vi "Read DI.vi"(6 "wait for reply (T)":bool=TRUE, 8 "error in":errorcluster, 11 "Module ID":i32=-1) -> (0 "error out":errorcluster, 1 "timed out?":bool, 3 "DI":bool[](array[boolean]))   [LabVIEW 2020, in "NI DAQ Aug 25.lvlib"]
doc: "Reads single or multiple DIs."
uses:
  NI DAQ Aug 25.lvlib
  Read DI Argument--cluster.ctl
  Read DI (Reply Payload)--cluster.ctl
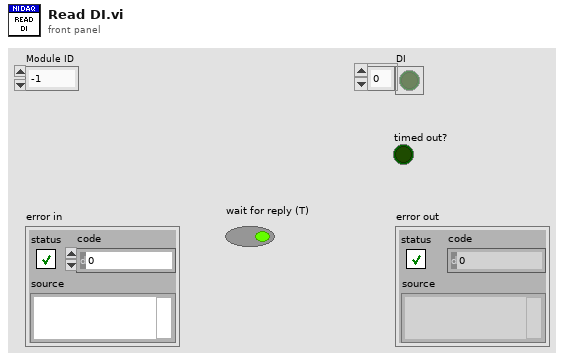
[diagram p1: front panel]
types:
  T1 = typedef "NI DAQ Aug 25.lvlib/Read DI Argument--cluster.ctl" = cluster{"Module ID":i32, "Boolean":bool, "Wait Notifier":refnum<notifier>, "wait for reply":bool}
  T2 = typedef "NI DAQ Aug 25.lvlib/Request Events--cluster.ctl" = cluster{"Stop Module":refnum<user-event>, "Show Panel":refnum<user-event>, "Hide Panel":refnum<user-event>, "Show Diagram":refnum<user-event>, "Get Module Execution Status":refnum<user-event>, "Draw FP in subpanel":refnum<user-event>, "Remove from subpanel":refnum<user-event>, "Set device name":refnum<user-event>, "Write DO":refnum<user-event>, "Create DO channel":refnum<user-event>, "Create DI channel":refnum<user-event>, "Read DI":refnum<user-event>}
  T3 = typedef "NI DAQ Aug 25.lvlib/Read DI (Reply Payload)--cluster.ctl" = cluster{"Module ID":i32, "error":errorcluster, "DI":bool[]}
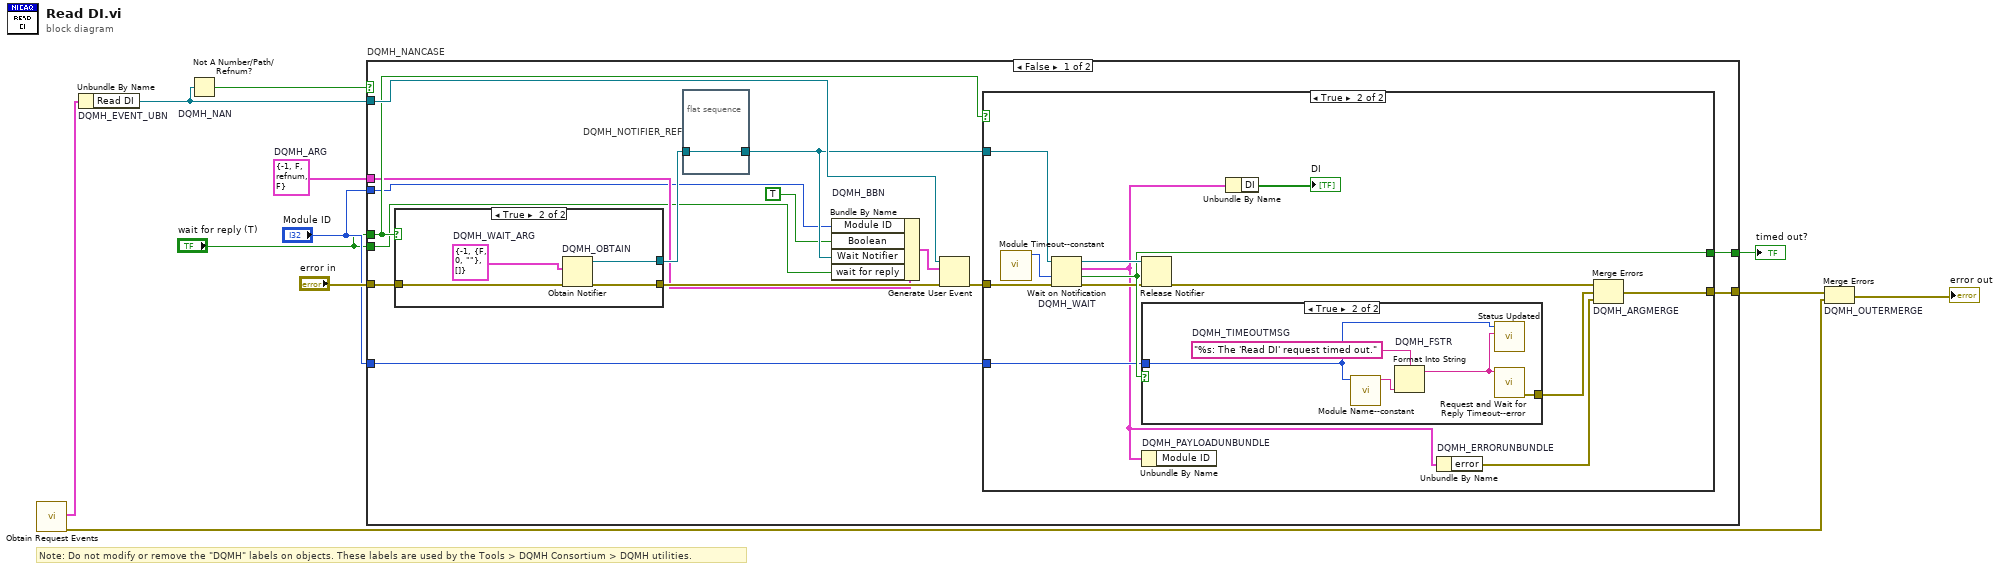
[diagram p0: block diagram]
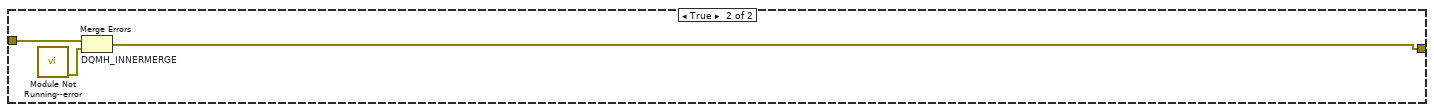
[diagram p5: hidden frame]
diagram:
  w5 = T1 {"Module ID"=-1, "Boolean"=FALSE, "Wait Notifier"=refnum, "wait for reply"=FALSE}  # DQMH_ARG
  # "Note: Do not modify or remove the \"DQMH\" labels on objects. These labels are used by the Tools > DQMH Consortium > DQMH utilities."
  n1 = call "Obtain Request Events.vi"() -> ("error out"=w2:errorcluster, "NI DAQ Aug 25 Request Events"=w1:T2)  [unwired: 10 in]
  n2 = Unbundle By Name "DQMH_EVENT_UBN"(w1) -> ("Read DI"=w6:refnum<user-event>)
  n3 = Not A Number/Path/Refnum? "DQMH_NAN"(number/path/refnum=w6) -> (NaN/Path/Refnum?=w7:bool)
  n4 = case "DQMH_NANCASE" shown="False" w7 {
    tunnel: "error in" -> [w26 w54]
    tunnel: w6 -> [w24 _]
    tunnel: [w21 w53] -> w8
    tunnel: [w22 _] -> w10
    tunnel: "wait for reply (T)" -> [w19 _]
    tunnel: w5 -> [w16 _]
    tunnel: "Module ID" -> [w15 _]
    tunnel: "Module ID" -> [w13 _]
    tunnel: "wait for reply (T)" -> [w12 _]
    frame False {
      n5 = case shown="True" w19 {
        tunnel: w26 -> [w47 w51]
        tunnel: [w47 w50] -> w23
        tunnel: [_ w48] -> w18
        frame False {
        }
        frame True {
          w49 = T3 {"Module ID"=-1, "error"={"status"=FALSE, "code"=0, "source"=""}, "DI"=[]}  # DQMH_WAIT_ARG
          n6 = Obtain Notifier "DQMH_OBTAIN"(notification data type=w49, error in (no error)=w51) -> (notifier out=w48:refnum<notifier>, error out=w50:errorcluster)  [unwired: 2 in, 1 out]
        }
      }
      n7 = flat-sequence "DQMH_NOTIFIER_REF" {
        tunnel: w18 -> [w27]
        tunnel: [w27] -> w17
        frame #0 {
        }
      }
      n8 = Bundle By Name "DQMH_BBN"(cluster=w16, "Module ID"=w15, "Boolean"=TRUE, "Wait Notifier"=w17, "wait for reply"=w12) -> (w20:T1)
      n9 = Generate User Event(user event=w24, event data cluster=w20, error in=w23) -> (error out=w25:errorcluster)  [unwired: 1 in, 1 out]
      n10 = case shown="True" w19 {
        tunnel: w25 -> [w28 w41]
        tunnel: w17 -> [_ w40]
        tunnel: [_ w38] -> w22
        tunnel: [w28 w37] -> w21
        tunnel: w13 -> [_ w31]
        frame False {
        }
        frame True {
          n11 = call "Module Timeout--constant.vi"() -> ("Module Timeout"=w32:i32)  [unwired: 11 in]
          n12 = Wait on Notification "DQMH_WAIT"(notifier=w40, timeout in ms (-1)=w32, error in (no error)=w41) -> (notifier out=w39:refnum<notifier>, notification=w30:T3, timed out?=w38:bool, error out=w36:errorcluster)  [unwired: 1 in]
          n13 = Release Notifier(notifier=w39, error in (no error)=w36) -> (error out=w35:errorcluster)  [unwired: 1 in, 2 out]
          n14 = case shown="True" w38 {
            tunnel: [_ w44] -> w33
            tunnel: w31 -> [_ w42]
            frame False {
            }
            frame True {
              w46 = "%s: The 'Read DI' request timed out."  # DQMH_TIMEOUTMSG
              n15 = call "Module Name--constant.vi"("Module ID"=w42) -> ("Module Name"=w43:string)  [unwired: 10 in]
              n16 = Format Into String "DQMH_FSTR"(format string=w46, w43) -> (resulting string=w45:string)  [unwired: 2 in, 1 out]
              n17 = call "Status Updated.vi"("Status"=w45, "Module ID"=w42) -> ()  [unwired: 9 in, 1 out]
              n18 = call "Request and Wait for Reply Timeout--error.vi"("Error Message"=w45) -> ("error out"=w44:errorcluster)  [unwired: 10 in]
            }
          }
          n19 = Unbundle By Name "DQMH_PAYLOADUNBUNDLE"(w30) -> ()  [unwired: 1 out]
          n20 = Unbundle By Name(w30) -> ("DI"=→"DI":bool[])
          n21 = Unbundle By Name "DQMH_ERRORUNBUNDLE"(w30) -> ("error"=w34:errorcluster)
          n22 = Merge Errors "DQMH_ARGMERGE"(w35, w33, w34) -> (w37:errorcluster)
        }
      }
    }
    frame True {
      n23 = call "Module Not Running--error.vi"() -> ("error out"=w52:errorcluster)  [unwired: 11 in]
      n24 = Merge Errors "DQMH_INNERMERGE"(w54, w52) -> (w53:errorcluster)
    }
  }
  "timed out?" <- w10
  n25 = Merge Errors "DQMH_OUTERMERGE"(w8, w2) -> (→"error out":errorcluster)
